vi "移动.vi"(3 "移动前":u16[][](array[numeric])=[[0, 0, 6, 1], [0, 0, 2, 0], [0, 0, 0, 0], [0, 0, 0, 1]], 4 "移动方式":string) -> (0 "移动后":i32[][](array[numeric]), 1 "分数":ext)   [LabVIEW 2020]
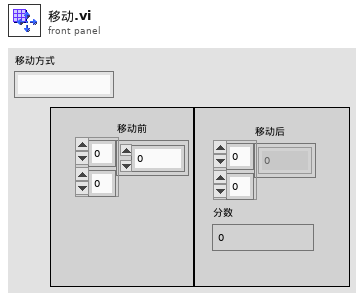
[diagram p1: front panel]
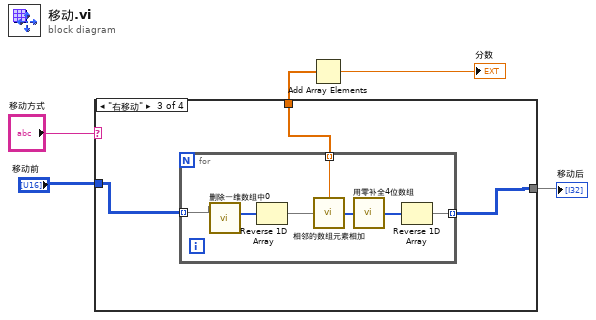
[diagram p0: block diagram]
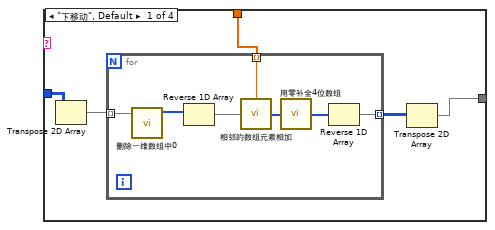
[diagram p2: hidden frame]
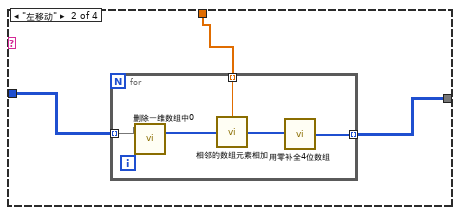
[diagram p3: hidden frame]
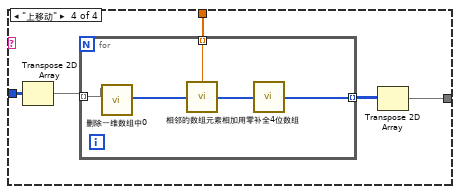
[diagram p4: hidden frame]
diagram:
  n1 = case shown="\"右移动\"" "移动方式" {
    tunnel: "移动前" -> [w6 w20 w28 w40]
    tunnel: [w8 w19 w26 w37] -> w4
    tunnel: [w7 w18 w27 w36] -> w3
    frame "下移动", Default {
      n2 = Transpose 2D Array(2D array=w6) -> (transposed array=w10:u16[][])
      n3 = for {
        tunnel: w10 -> [w12] mode=indexing
        tunnel: [w15] -> w9 mode=indexing
        tunnel: [w13] -> w7 mode=indexing
        n4 = call "删除一维数组中0.vi"("数组输入"=w12) -> ("数组输出"=w11:u16[])  [unwired: 10 in]
        n5 = Reverse 1D Array(array=w11) -> (reversed array=w16:u16[])
        n6 = call "相邻的数组元素相加.vi"("数组输入"=w16) -> ("数组输出"=w17:i32[], "分数"=w13:ext)  [unwired: 2 in]
        n7 = call "用零补全4位数组.vi"("数组输入"=w17) -> ("数组输出"=w14:i32[])
        n8 = Reverse 1D Array(array=w14) -> (reversed array=w15:i32[])
      }
      n9 = Transpose 2D Array(2D array=w9) -> (transposed array=w8:i32[][])
    }
    frame "左移动" {
      n10 = for {
        tunnel: w20 -> [w21] mode=indexing
        tunnel: [w25] -> w19 mode=indexing
        tunnel: [w23] -> w18 mode=indexing
        n11 = call "删除一维数组中0.vi"("数组输入"=w21) -> ("数组输出"=w22:u16[])  [unwired: 10 in]
        n12 = call "相邻的数组元素相加.vi"("数组输入"=w22) -> ("数组输出"=w24:i32[], "分数"=w23:ext)  [unwired: 2 in]
        n13 = call "用零补全4位数组.vi"("数组输入"=w24) -> ("数组输出"=w25:i32[])
      }
    }
    frame "右移动" {
      n14 = for {
        tunnel: w28 -> [w30] mode=indexing
        tunnel: [w33] -> w26 mode=indexing
        tunnel: [w31] -> w27 mode=indexing
        n15 = call "删除一维数组中0.vi"("数组输入"=w30) -> ("数组输出"=w29:u16[])  [unwired: 10 in]
        n16 = Reverse 1D Array(array=w29) -> (reversed array=w34:u16[])
        n17 = call "相邻的数组元素相加.vi"("数组输入"=w34) -> ("数组输出"=w35:i32[], "分数"=w31:ext)  [unwired: 2 in]
        n18 = call "用零补全4位数组.vi"("数组输入"=w35) -> ("数组输出"=w32:i32[])
        n19 = Reverse 1D Array(array=w32) -> (reversed array=w33:i32[])
      }
    }
    frame "上移动" {
      n20 = Transpose 2D Array(2D array=w40) -> (transposed array=w39:u16[][])
      n21 = for {
        tunnel: w39 -> [w41] mode=indexing
        tunnel: [w45] -> w38 mode=indexing
        tunnel: [w43] -> w36 mode=indexing
        n22 = call "删除一维数组中0.vi"("数组输入"=w41) -> ("数组输出"=w42:u16[])  [unwired: 10 in]
        n23 = call "相邻的数组元素相加.vi"("数组输入"=w42) -> ("数组输出"=w44:i32[], "分数"=w43:ext)  [unwired: 2 in]
        n24 = call "用零补全4位数组.vi"("数组输入"=w44) -> ("数组输出"=w45:i32[])
      }
      n25 = Transpose 2D Array(2D array=w38) -> (transposed array=w37:i32[][])
    }
  }
  "移动后" <- w4
  n26 = Add Array Elements(numeric array=w3) -> (sum=→"分数":ext)
